vi "Wysyllanie danych do PC  2.vi"(5 "remote port":u16, 6 "output cluster":cluster{"CAN frame":T1, "Delay":dbl} {"CAN frame"."type" items=["CAN Data", "CAN Remote"]; "CAN frame"."identifier" format="%.0x"}, 7 "adres":u32, 8 "error in (no error)":errorcluster, 11 "UDP Network Connection in":refnum<k16>) -> (0 "error out":errorcluster, 3 "UDP Network Connection out":refnum<k16>)   [LabVIEW 2015]
uses:
  <vilib>/RioEmbeddedCAN/RioEmbeddedCAN.llb/CANFrameControl.ctl
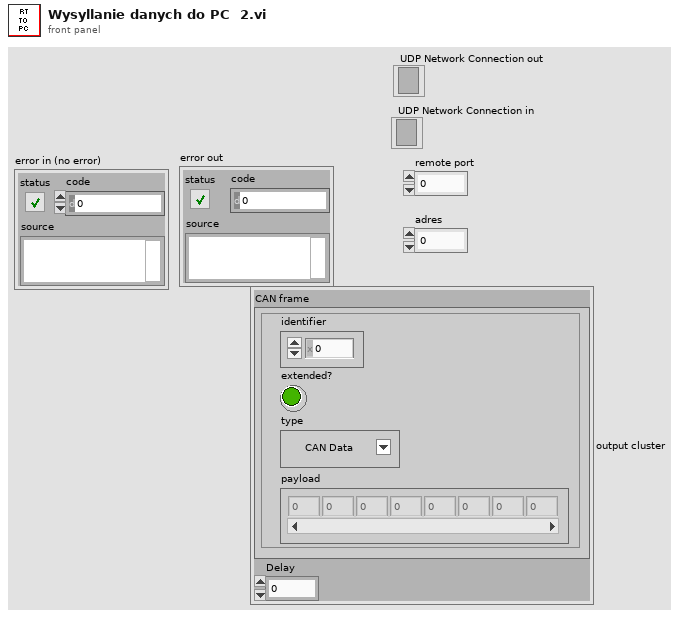
[diagram p1: front panel]
types:
  T1 = typedef "CANFrameControl.ctl" = cluster{"identifier":u32, "extended?":bool, "type":u8, "payload":u8[]}
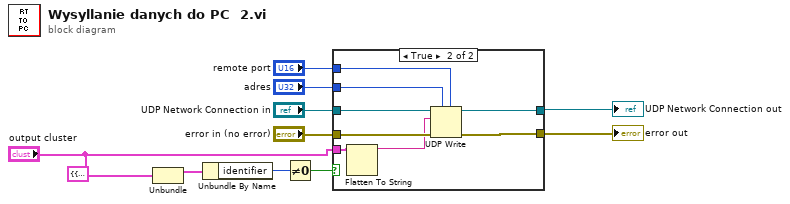
[diagram p0: block diagram]
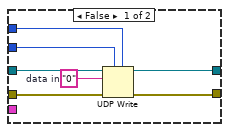
[diagram p2: hidden frame]
diagram:
  (unwired) cluster{"CAN frame":T1, "Delay":dbl} {"CAN frame"={"identifier"=0, "extended?"=FALSE, "type"=0, "payload"=[]}, "Delay"=0.0} ("output cluster")
  n1 = Unbundle("output cluster") -> ("CAN frame"=w2:T1)  [unwired: 1 out]
  n2 = Unbundle By Name(w2) -> ("identifier"=w3:u32)
  n3 = Not Equal To 0?(x=w3) -> (x != 0?=w6:bool)
  n4 = case shown="True" w6 {
    tunnel: [w15 w25] -> w9
    tunnel: "adres" -> [w12 w24]
    tunnel: "remote port" -> [w11 w23]
    tunnel: "UDP Network Connection in" -> [w17 w22]
    tunnel: "error in (no error)" -> [w16 w21]
    tunnel: [w14 w20] -> w10
    tunnel: "output cluster" -> [_ w19]
    frame False {
      w13 = "0"  # data in
      n5 = UDP Write(address=w12, port or service name=w11, connection ID=w17, data in=w13, 8:w16) -> (error out=w14:errorcluster, 3:w15:refnum<k16>)  [unwired: 1 in]
    }
    frame True {
      n6 = Flatten To String(anything=w19) -> (data string=w18:string)  [unwired: 3 in, 2 out]
      n7 = UDP Write(address=w24, port or service name=w23, connection ID=w22, data in=w18, 8:w21) -> (error out=w20:errorcluster, 3:w25:refnum<k16>)  [unwired: 1 in]
    }
  }
  "error out" <- w10
  "UDP Network Connection out" <- w9
